vi "RSZVB Set Mixer Delay Correction.vi"(8 "error in (no error)":errorcluster {"code" format="%.0x"}, 9 "Correction (Off)":bool, 10 "Channel (1)":i32=1, 11 "VISA session":refnum<visa-resource-name>) -> (0 "error out":errorcluster {"code" format="%.0x"}, 3 "dup VISA session":refnum<visa-resource-name>)   [LabVIEW 2011]
doc: "Qualifies whether the analyzer applies the current mixer delay meas. calibration data. \n\nNotes:\n\n(1) This VI requires options R&S ZVA-K9 and R&S ZVA-K4.\n\nRemote-control command(s):\n[SENSe<Ch>:]FREQuency:MDELay:CORRection[:STATe]"
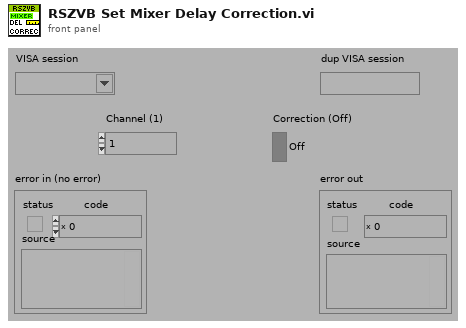
[diagram p1: front panel]
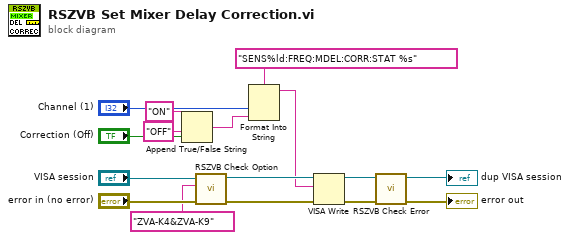
[diagram p0: block diagram]
diagram:
  n1 = Append True/False String(1:"Correction (Off)", 2:"OFF" ("false string"), 3:"ON" ("true string")) -> (0:w8:string)  [unwired: 1 in]
  n2 = call "RSZVB Check Option.vi"("error in (no error)"="error in (no error)", "Options"="ZVA-K4&ZVA-K9", "VISA session"="VISA session") -> ("error out"=w7:errorcluster, "dup VISA session"=w6:refnum<visa-resource-name>)  [unwired: 7 in]
  n3 = Format Into String(format string="SENS%ld:FREQ:MDEL:CORR:STAT %s", "Channel (1)", w8) -> (resulting string=w5:string)  [unwired: 2 in, 1 out]
  n4 = VISA Write(VISA resource name=w6, write buffer=w5, error in (no error)=w7) -> (VISA resource name out=w3:refnum<visa-resource-name>, error out=w4:errorcluster)  [unwired: 1 out]
  n5 = call "RSZVB Check Error.vi"("error in (no error)"=w4, "VISA session"=w3) -> ("error out"=→"error out":errorcluster, "dup VISA session"=→"dup VISA session":refnum<visa-resource-name>)  [unwired: 8 in]
